vi "Run.vi"(7 "Stop Demo":refnum<user-event>, 8 "error in":errorcluster, 9 "Try It Button":refnum<vi>, 10 "Main Subpanel":refnum<vi>, 11 "Passive in":refnum<class "Passive.lvclass">) -> (0 "error out":errorcluster, 3 "Passive out":refnum<class "Passive.lvclass">)   [LabVIEW 2020, in "Passive.lvclass"]
uses:
  Passive.lvclass
  Demo_class/Demo.lvclass
  Passive.lvclass/Passive.ctl
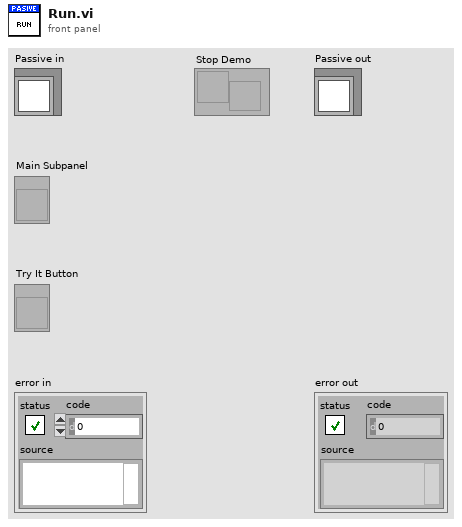
[diagram p1: front panel]
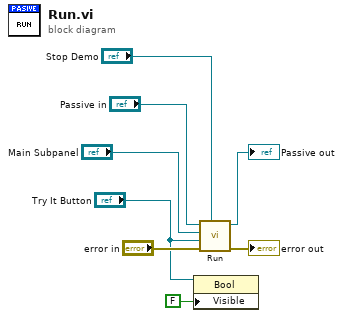
[diagram p0: block diagram]
diagram:
  n1 = property class="Bool"(reference="Try It Button", "Visible"=FALSE) -> ()  [unwired: 1 in, 2 out]
  n2 = call-parent "Run.vi"("Stop Demo"="Stop Demo", "error in"="error in", "Try It Button"="Try It Button", "Main Subpanel"="Main Subpanel", "Demo in"="Passive in") -> ("error out"=→"error out":errorcluster, "Demo out"=→"Passive out":refnum<class "Passive.lvclass">)  [unwired: 4 in, 1 out]
